vi "ApplicationConfigCreateIniFile.vi"(8 "error in (no error)":errorcluster, 11 "Nom Fichier ini":path) -> (0 "error out":errorcluster)   [LabVIEW 2011]
uses:
  Ctrls/ApplicationConfig.ctl
  Ctrls/MessageHandlerConfig.ctl
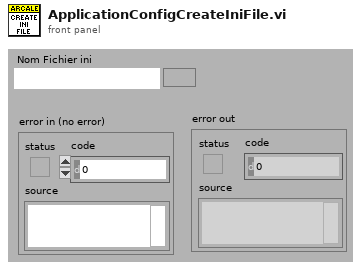
[diagram p1: front panel]
types:
  T1 = typedef "ApplicationConfig.ctl" = cluster{"Data Path":path, "MessageHandlerConfig":T2, "Simulation":bool, "Dictionnary":string}
  T2 = typedef "MessageHandlerConfig.ctl" = cluster{"Max log files":u32, "Max messages per file":u32}
  T3 = typedef "ApplicationInfos.ctl" = cluster{"ApplicationName":string, "ApplicationVersion":string, "Logo 600X200 path":path, "Logo 400X400 path":path, "Client":string}
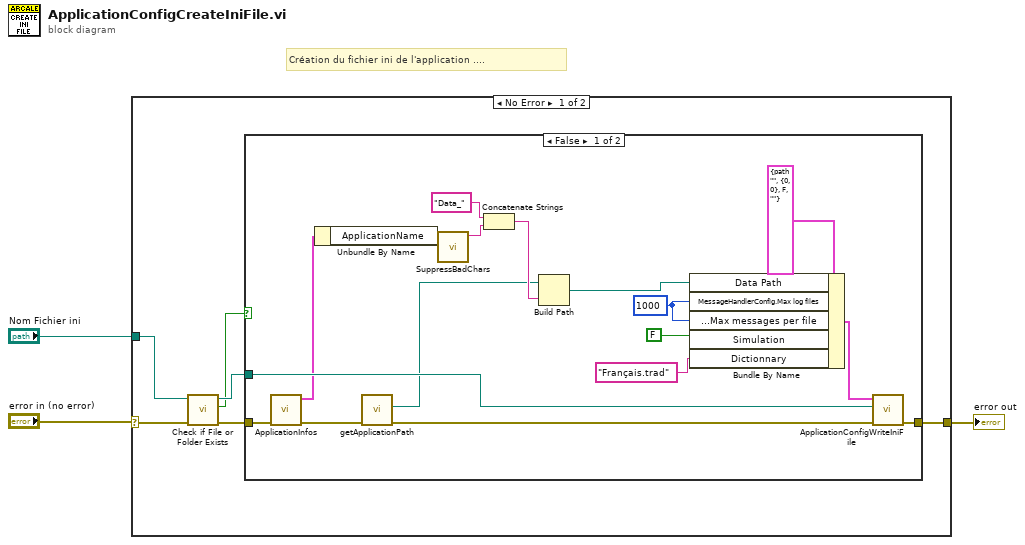
[diagram p0: block diagram]
diagram:
  # "Création du fichier ini de l'application ...."
  n1 = case shown="No Error" "error in (no error)" {
    selector: "error in (no error)" -> [w6 w28]
    tunnel: [w8 w28] -> w2
    tunnel: "Nom Fichier ini" -> [w9 _]
    frame No Error {
      n2 = call <vilib>:"Check if File or Folder Exists.vi"("error in (no error)"=w6, "path"=w9) -> ("error out"=w5:errorcluster, "file or folder exists?"=w4:bool, "dup path"=w7:path)  [unwired: 7 in]
      n3 = case shown="False" w4 {
        tunnel: [w25 w27] -> w8
        tunnel: w7 -> [w21 _]
        tunnel: w5 -> [w20 w27]
        frame False {
          w23 = u32 1000 ("MessageHandlerConfig.Max log files")
          n4 = call "ApplicationInfos.vi"("error in (no error)"=w20) -> ("error out"=w11:errorcluster, "ApplicationInfo"=w19:T3)  [unwired: 9 in]
          n5 = Unbundle By Name(w19) -> ("ApplicationName"=w18:string)
          n6 = call "getApplicationPath.vi"("error in (no error)"=w11) -> ("error out"=w10:errorcluster, "ApplicationPath"=w12:path)  [unwired: 9 in]
          n7 = call "SuppressBadChars.vi"("StringIn"=w18) -> ("StringOut"=w16:string)  [unwired: 9 in, 1 out]
          n8 = Concatenate Strings("Data_", w16) -> (w15:string)
          n9 = Build Path(base path=w12, name or relative path=w15) -> (appended path=w14:path)
          n10 = Bundle By Name(cluster=T1 {"Data Path"=path "", "MessageHandlerConfig"={"Max log files"=0, "Max messages per file"=0}, "Simulation"=FALSE, "Dictionnary"=""} ("ApplicationConfig"), "Data Path"=w14, "MessageHandlerConfig.Max log files"=w23, "MessageHandlerConfig.Max messages per file"=w23, "Simulation"=FALSE, "Dictionnary"="Français.trad" ("name or relative path")) -> (w24:T1)
          n11 = call "ApplicationConfigWriteIniFile.vi"("error in (no error)"=w10, "IniFilePath"=w21, "ApplicationConfig"=w24) -> ("error out"=w25:errorcluster)  [unwired: 8 in]
        }
        frame True {
        }
      }
    }
    frame Error {
    }
  }
  "error out" <- w2
